vi "New dotNET TCP Socket from Reference.vi"(8 "error in (no error)":errorcluster, 11 "TcpClient":refnum<k24>) -> (0 "error out":errorcluster, 3 "dotNET TCP Socket out":refnum<class "dotNET TCP Socket.lvclass">)   [LabVIEW 2013, in "dotNET SSL Socket.lvlib" / "dotNET TCP Socket.lvclass"]
doc: "Creates new dotNET TCP object from a .NET TCPClient reference."
uses:
  dotNET TCP Socket.lvclass
  dotNET TCP Socket.lvclass/dotNET TCP Socket.ctl
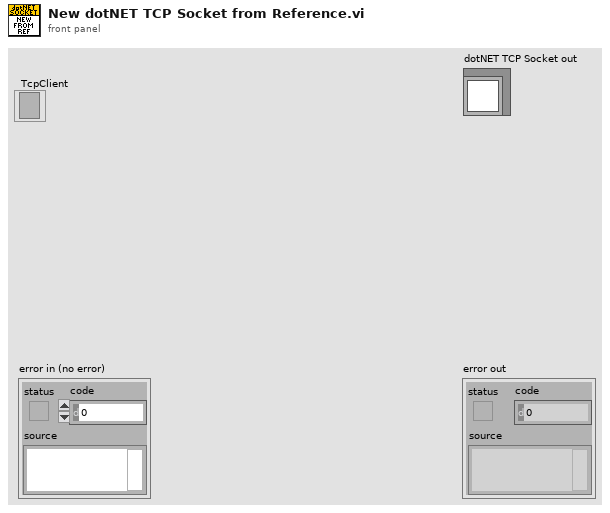
[diagram p1: front panel]
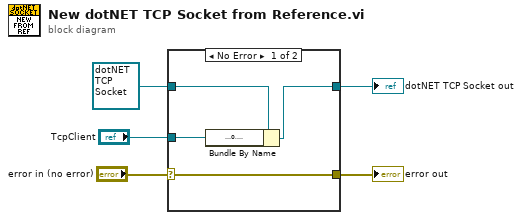
[diagram p0: block diagram]
diagram:
  n1 = case shown="No Error" "error in (no error)" {
    selector: "error in (no error)" -> [w9 w11]
    tunnel: [w9 w11] -> w4
    tunnel: [w7 w10] -> w3
    tunnel: refnum<class "dotNET TCP Socket.lvclass"> refnum ("dotNET TCP Socket in") -> [w8 w10]
    tunnel: "TcpClient" -> [w6 _]
    frame No Error {
      n2 = Bundle By Name(cluster=w8, "TcpClient"=w6) -> (w7:refnum<class "dotNET TCP Socket.lvclass">)
    }
    frame Error {
    }
  }
  "error out" <- w4
  "dotNET TCP Socket out" <- w3
